vi "trace_properties_string.vi"(0 "reference in":refnum<class "OSA.lvclass">, 2 "property":T4, 3 "dataType":T3, 4 "trace idx":u32, 5 "error in (no error)":errorcluster) -> (14 "reference out":refnum<class "OSA.lvclass">, 16 "property out":T2, 17 "property out array":T1(array[cluster]), 19 "error out":errorcluster)   [LabVIEW 2010, in "OSA.lvclass"]
doc: "Trace properties returned as string."
uses:
  OSA.lvclass
  typeDef/trace_properties_string.ctl
  typeDef/acq_dataType.ctl
  FTSLib.dll
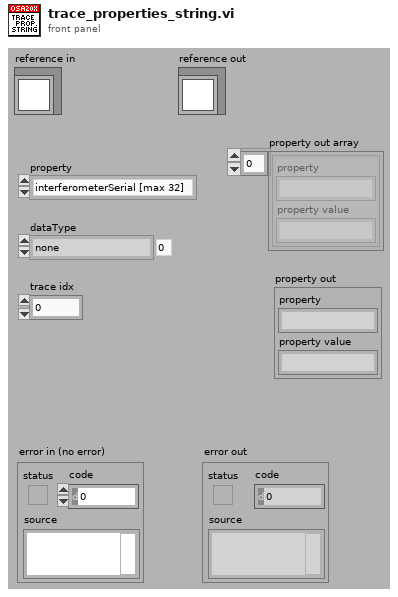
[diagram p1: front panel]
types:
  T1 = cluster{"property":string, "property value":string}[]
  T2 = cluster{"property":string, "property value":string}
  T3 = typedef "OSA.lvclass/acq_dataType.ctl" = enum16{"none", "interferogram", "spectrum"}
  T4 = typedef "OSA.lvclass/trace_properties_string.ctl" = enum16{"interferometerSerial [max 32]", "name [max 32]", "comment [max 128]", "source [max 24]", "instr_operator [max 24]", "instr_model_str [max 24]", "all_stringParameters"}
  T5 = typedef "OSA.lvclass/ObjectAttributes.ctl" = cluster{"Stop":bool, "dataType":T3, "spectrometerIdx":u16, "buffer size interferogram":i32, "interferogram":cluster{"new":bool, "plot_x_ min":sgl, "plot_x_max":sgl, "plot_y_min":sgl, "plot_y_max":sgl, "Graph Intrfrgrm":T6, "timeStamp":u32, "signal (%)":dbl, "traces":cluster{"idx":u32, "broadBand":bool, "monoChromatic":bool, "peakToPeakSignal":dbl, "peakToPeakPos":dbl}[], "traces idx last":i32}, "spectrum":cluster{"new":bool, "plot_x_min":sgl, "plot_x_max":sgl, "plot_unit_x":T7, "plot_unit_y":T8, "plot_y_min":sgl, "plot_y_max":sgl, "Graph Spectrum":T6, "timeStamp":u32, "X_VAL_OPTIONS":enum16{"MIN_MAX", "ARRAY"}, "traces":cluster{"idx":u32}[], "traces idx last":i32}, "Thorlabs_OSA_64.lvclass:queue_action.ctlqueue ref":refnum<queue>, "action":T9, "plot zoom step":dbl, "buffer semaphore":T10, "acq stopped":bool, "dataType active":T3, "temperature (degr C)":sgl, "pressure (hPa)":sgl, "rel humidity (%)":sgl, "settings":cluster{"resolution":T11, "sensitivity":T12, "Average":bool, "average nr":u32, "apodisation":T13, "acq delay (ms)":u32, "airMesure":T14, "wmtr on":bool, "intfgrm_smooth_width":u16, "intfgrm_smooth_nrOfPasses":u16, "intfgrm_smooth":T15, "phaseCorrection":T16, "zeroFill":u8, "spectr_smooth":T15, "spectr_smooth_width":u16, "spectr_smooth_nrOfPasses":u16, "resolution (/cm)":sgl, "REF wavelength, (nm)":dbl, "gain_idx":u16, "gainAuto":bool, "gain_relative":dbl, "PD sensitivity mode":T17, "PD senseMode implemented":bool, "SensorTemperature implemented":bool, "SensorPressure implemented":bool, "SensorHumidity implemented":bool}, "peaks position":sgl[], "peaks width":sgl[], "peaks height":sgl[], "peaks max nr":u32, "peaks latest nr":i32, "peaks new":bool, "power":dbl, "power new":bool, "path":string, "wavelength (WNr)":dbl, "wavelength new":bool, "buffer size spectrum":i32, "status":string, "VI reference":refnum<vi>, "funcPointer":u64, "libraryPointer":u64, "singleAcquisition":bool, "coherenceLength (cm)":dbl, "coherenceLength new":bool, "spectrometer model":string, "spectrometer serial nr":string, "peaks thld left":sgl[], "peaks thld right":sgl[], "coherenceLength error (cm)":dbl, "ADC bits":u16, "peaks position centroid":sgl[], "peaks height centroid":sgl[], "OSA series":T18, "channel index spectrum":u16, "spectrometer rangeLow, (/cm)":dbl, "spectrometer rangeHigh, (/cm)":dbl, "channel index interferogram":u16}
  T6 = typedef "OSA.lvclass/graph_intensity.ctl" = refnum<vi>
  T7 = typedef "OSA.lvclass/spectrum_x_unit.ctl" = enum16{"wavenr/cm", "THz", "eV", "nm_air", "nm_vac"}
  T8 = typedef "OSA.lvclass/y_unit.ctl" = enum16{"ADC counts", "dBm pwr absolute", "dBm pwr density", "mW pwr absolute", "mW pwr density"}
  T9 = typedef "OSA.lvclass/queue_action.ctl" = enum16{"none", "stop", "GUI_plotInterferogram", "GUI_plotSpectrum", "GUI_plotInterferogramRescale", "GUI_plotSpectrumRescale", "GUI_plotInterferogramReset", "GUI_plotSpectrumReset", "GUI_plotInterferogramAutoScaleY", "GUI_plotSpectrumAutoScaleY", "GUI_plotInterferogramZoomOut", "GUI_plotSpectrumZoomOut", "GUI_plotInterferogramPane", "GUI_plotSpectrumPane", "GUI_plotInterferogramZoomMouse", "GUI_plotSpectrumZoomMouse", "ENVIRONMENT temperature", "ENVIRONMENT pressure", "MODE_resolution set", "MODE_resolution get", "MODE_sensitivity set", "MODE_sensitivity get", "MODE_PDTemperature set", "MODE_PDTemperature get", "REBOOT/RESET firmware", "ACQASYNC_acquireSingleSpectrum", "ACQASYNC_continuous start", "ACQASYNC_continuous stop\n", "ACQASYNC_get last interferogram", "ACQASYNC_get last spectrum", "ACQASYNC_get last waveNr", "ACQOPT_interferogram smoothing set", "ACQOPT_interferogram smoothing get", "ACQOPT_spectrum smoothing set", "ACQOPT_spectrum smoothing get", "ACQOPT_apodisation type set", "ACQOPT_apodisation type get", "ACQOPT_phase correction type set", "ACQOPT_phase correction type get", "ACQOPT_acqIntervall_set", "ACQOPT_acqIntervall_get", "ACQOPT_average spectrum set", "ACQOPT_average spectrum get", "ACQOPT_rolling average set", "ACQOPT_rolling average get", "ACQOPT_zero fill factor set", "ACQOPT_zero fill factor get", "ACQOPT_cycle counting set", "ACQOPT_cycle counting get", "ACQOPT_air measure option set", "ACQOPT_air measure option get", "ACQOPT_gainLevel auto get", "ACQOPT_gainLevel auto set", "ACQOPT_gainLevel get", "ACQOPT_gainLevel set", "ACQOPT_getAll", "INSTRUMENT_PROPERTY_range_WaveNr_min", "INSTRUMENT_PROPERTY_range_WaveNr_max", "INSTRUMENT_PROPERTY_reference_wavelength_cm^-1", "INSTRUMENT_PROPERTY_samplesPerRefPeriod", "INSTRUMENT_PROPERTY_resolution_waveNrPercm", "INSTRUMENT_PROPERTY_availableGainLevels", "INSTRUMENT_PROPERTY_status", "CONVERT", "ANALYSE_POWER", "ANALYSE_PEAKS", "ANALYSE_WAVELENGTH", "ANALYSE_SPECTRUM", "ANALYSE_INTERFEROGRAM", "ANALYSE_COHERENCE_LENGTH", "MATH", "MATH_power", "MATH_peaks", "FILE", "miscellaneous"}
  T10 = typedef "Semaphore RefNum" = refnum<k1>
  T11 = typedef "OSA.lvclass/resolution.ctl" = enum16{"low", "high"}
  T12 = typedef "OSA.lvclass/sensitivityMode.ctl" = enum16{"low", "low medium", "high medium", "high"}
  T13 = typedef "OSA.lvclass/apodisation.ctl" = enum16{"NONE", "NORTON_BEER_WEAK", "NORTON_BEER_MEDIUM", "NORTON_BEER_STRONG", "TRIANGULAR", "COSINE", "HANN", "HAMMING", "BLACKMANHARRIS3", "BLACKMANHARRIS4", "GAUSSIAN"}
  T14 = typedef "OSA.lvclass/airMeasure.ctl" = enum16{"TEMPERATURE", "PRESSURE"}
  T15 = typedef "OSA.lvclass/smoothing.ctl" = enum16{"NONE", "BINOMIAL", "SAVITSKY_GOLAY", "FOURIER", "MOVING_AVERAGE", "GAUSSIAN"}
  T16 = typedef "OSA.lvclass/phaseCorrection.ctl" = enum16{"NONE", "MERTZ", "FORMAN", "MERTZ_FILE", "FORMAN_FILE", "FUTURE COMP."}
  T17 = typedef "OSA.lvclass/PDTemperatureMode.ctl" = enum16{"cool: better sensitivity/noise floor", "warm: extended wl range"}
  T18 = typedef "OSA.lvclass/OSA_series.ctl" = enum16{"OSA200", "OSA300", "UNKNOWN"}
  T19 = cluster{"idx":u32, "broadBand":bool, "monoChromatic":bool, "peakToPeakSignal":dbl, "peakToPeakPos":dbl}[]
  T20 = enum16{"interferometerSerial [max 32]", "name [max 32]", "comment [max 128]", "source [max 24]", "instr_operator [max 24]", "instr_model_str [max 24]", "all_stringParameters"}
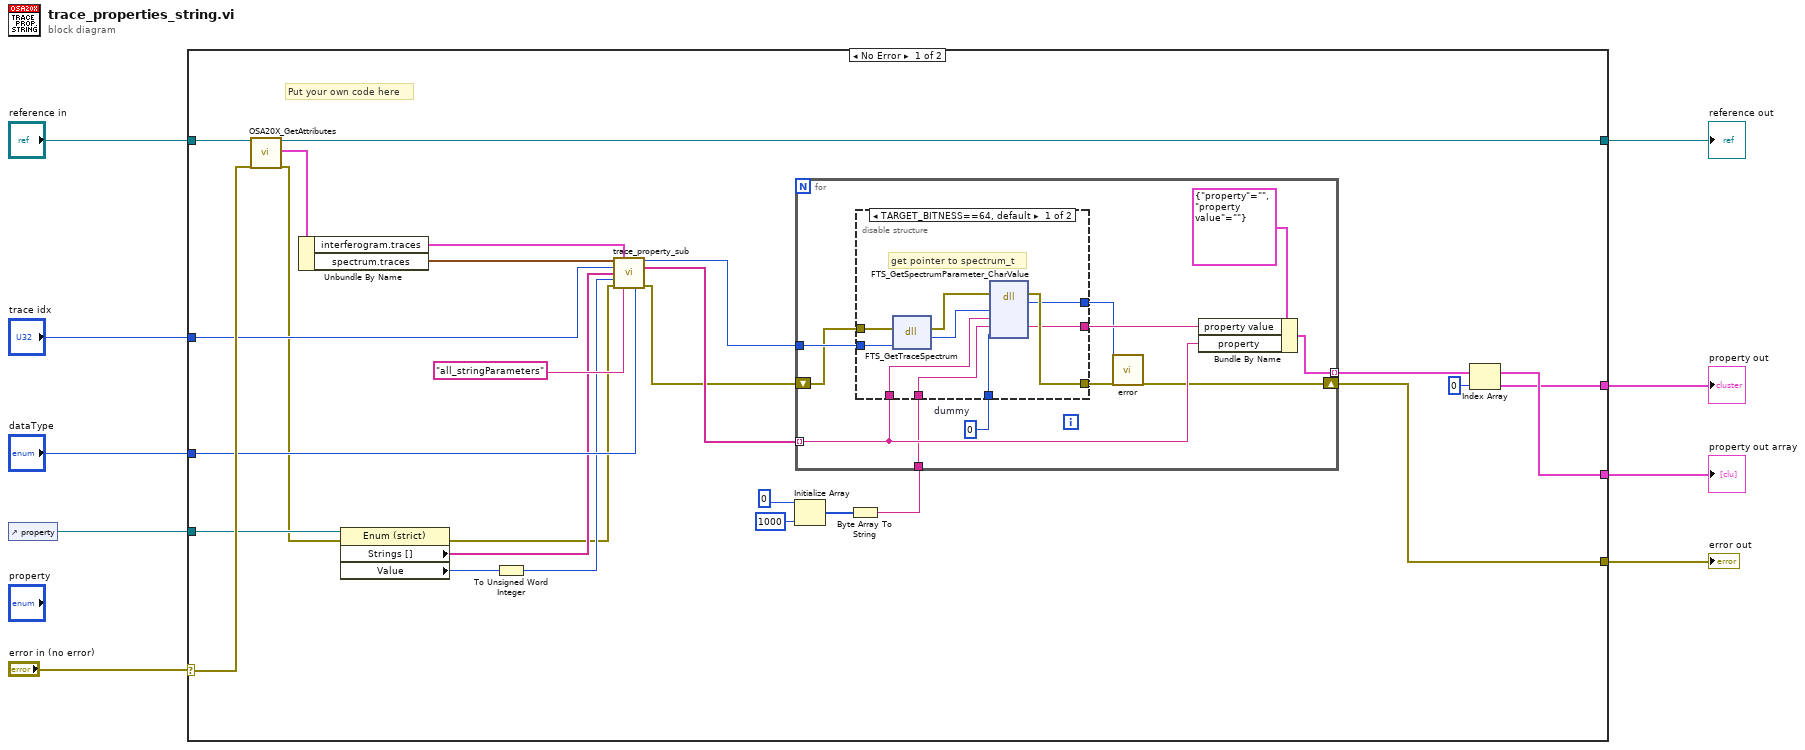
[diagram p0: block diagram]
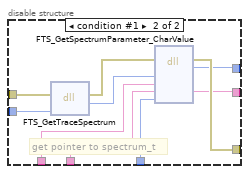
[diagram p2: hidden frame]
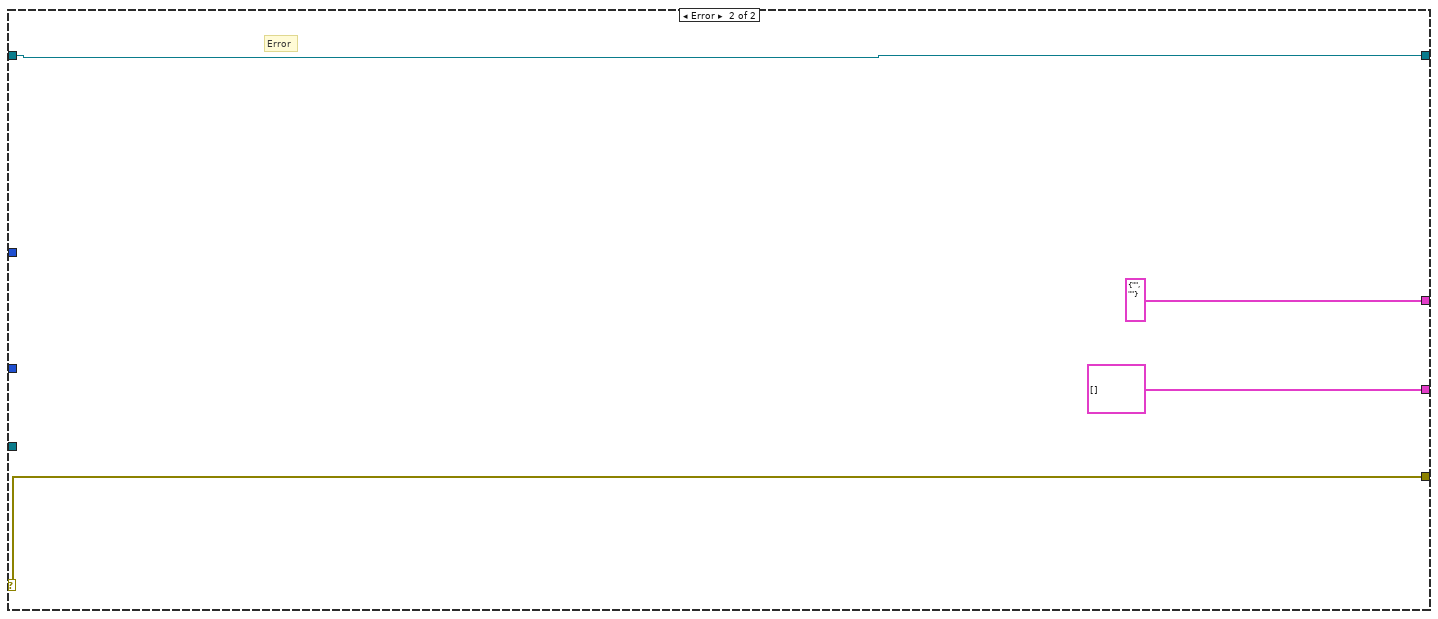
[diagram p3: hidden frame]
diagram:
  n1 = control-ref of="property"() -> (w3:refnum<vi>)
  n2 = case shown="No Error" "error in (no error)" {
    selector: "error in (no error)" -> [w34 w70]
    tunnel: [w31 w70] -> w9
    tunnel: "reference in" -> [w33 w69]
    tunnel: [w32 w69] -> w6
    tunnel: "dataType" -> [w23 _]
    tunnel: [w30 T1 []] -> w1
    tunnel: "trace idx" -> [w25 _]
    tunnel: w3 -> [w19 _]
    tunnel: [w28 T2 {"property"="", "property value"=""}] -> w2
    frame No Error {
      # "Put your own code here"
      n3 = call "OSA20X_GetAttributes.vi"("reference in"=w33, "error in (no error)"=w34) -> ("reference out"=w32:refnum<class "OSA.lvclass">, "Data"=w35:T5, "error out"=w18:errorcluster)  [unwired: 14 in, 1 out]
      n4 = Unbundle By Name(w35) -> ("interferogram.traces"=w27:T19, "spectrum.traces"=w26:cluster{"idx":u32}[])
      n5 = property class="Enum (strict)"(reference=w19, error in=w18) -> (error out=w14:errorcluster, "Strings []"=w17:string[], "Value"=w16:T20)  [unwired: 1 out]
      n6 = To Unsigned Word Integer(number=w16) -> (unsigned 16bit integer=w15:u16)
      n7 = call "trace_property_sub.vi"("traces_spectrum"=w26, "traces_interferogram"=w27, "trace idx"=w25, "Strings enum"=w17, "Value enum"=w15, "error in (no error)"=w14, "all string"="all_stringParameters" ("y"), "dataType"=w23) -> ("global trace idx"=w22:u32, "parameter names"=w21:string[], "error out"=w20:errorcluster)  [unwired: 4 in, 1 out]
      n8 = Initialize Array(u8 0 ("element"), 1000 ("dimension size")) -> (w11:u8[])
      n9 = Byte Array To String(unsigned byte array=w11) -> (string=w10:string)
      n10 = for {
        tunnel: w22 -> [w46]
        tunnel: [w43] -> w30 mode=indexing
        shift-right: [w37] -> w31
        shift-left: w20 -> [w45]
        tunnel: w21 -> [w42] mode=indexing
        tunnel: w10 -> [w40]
        w41 = u32 0  # dummy
        n11 = disable-structure shown="TARGET_BITNESS==64, default" {
          disable-tunnel: w46 -> [w56 w65]
          disable-tunnel: w45 -> [w53 w66]
          disable-tunnel: [w52 w63] -> w38
          disable-tunnel: w42 -> [w51 w61]
          disable-tunnel: w41 -> [w50 w59]
          disable-tunnel: w40 -> [w49 w60]
          disable-tunnel: [w48 w57] -> w39
          disable-tunnel: [w47 w58] -> w36
          frame condition #0 (active) {
            # "get pointer to spectrum_t"
            n12 = dll-call lib="FTSLib.dll" fn="FTS_GetTraceSpectrum"(error in=w53, "traceIdx"=w56) -> (error out=w54:errorcluster, "spectrum_t_pointer"=w55:u64)  [unwired: 3 in, 1 out]
            n13 = dll-call lib="FTSLib.dll" fn="FTS_GetSpectrumParameter_CharValue"(error in=w54, "spectrum_t_pointer"=w55, "parameter_name"=w51, "parameter_value"=w49, "array_index"=w50) -> (error out=w52:errorcluster, "returnVal"=w47:i32, "parameter_value"=w48:string)  [unwired: 5 in, 1 out]
          }
          frame condition #1 {
            # "get pointer to spectrum_t"
            n14 = dll-call lib="FTSLib.dll" fn="FTS_GetTraceSpectrum"(error in=w66, "traceIdx"=w65) -> (error out=w64:errorcluster, "spectrum_t_pointer"=w62:u32)  [unwired: 3 in, 1 out]
            n15 = dll-call lib="FTSLib.dll" fn="FTS_GetSpectrumParameter_CharValue"(error in=w64, "spectrum_t_pointer"=w62, "parameter_name"=w61, "parameter_value"=w60, "array_index"=w59) -> (error out=w63:errorcluster, "returnVal"=w58:i32, "parameter_value"=w57:string)  [unwired: 5 in, 1 out]
          }
        }
        n16 = call "error.vi"("result code"=w36, "error in (no error)"=w38) -> ("error out"=w37:errorcluster)  [unwired: 15 in, 2 out]
        n17 = Bundle By Name(cluster=T2 {"property"="", "property value"=""}, "property value"=w39, "property"=w42) -> (w43:T2)
      }
      n18 = Index Array(array=w30, index=0) -> (element=w28:T2)
    }
    frame Error {
      # "Error"
    }
  }
  "error out" <- w9
  "reference out" <- w6
  "property out" <- w2
  "property out array" <- w1
